vi "delete alarm comparison.vi"(8 "error in":errorcluster, 9 "compare index":i32, 10 "alarm name":string, 11 "alarms module configuration in":refnum<class "alarms module configuration.lvclass">) -> (0 "error out":errorcluster, 2 "removed channels":refnum<class "TBM channel.lvclass">[](array[class]), 3 "alarms module configuration out":refnum<class "alarms module configuration.lvclass">)   [LabVIEW 2013, in "alarms module configuration.lvclass"]
uses:
  alarms module configuration.lvclass
  <vilib>/NI/Tag Bus Module Framework/channel/TBM channel.lvclass
  alarms module configuration.lvclass/alarms module configuration.ctl
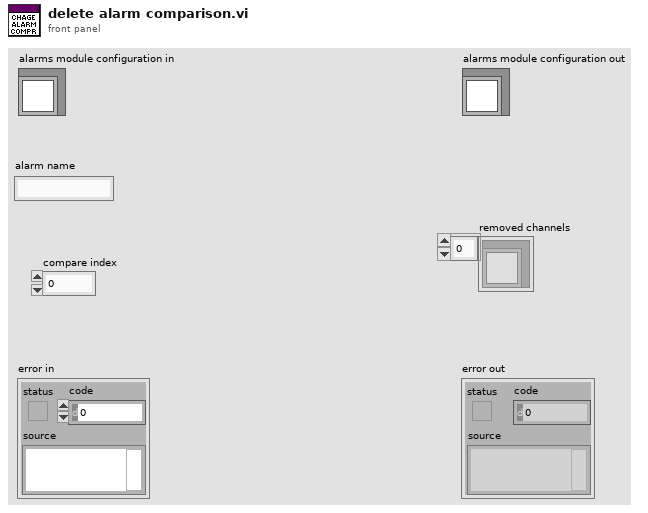
[diagram p1: front panel]
types:
  T1 = typedef "alarms module configuration.lvclass/alarm configuration.ctl" = cluster{"alarm name":string, "comparisons":T2[], "unlatch":refnum<class "TBM channel.lvclass">, "output":refnum<class "TBM channel.lvclass">, "boolean op":T4}
  T2 = typedef "alarms module configuration.lvclass/alarm comparison.ctl" = cluster{"input channel":refnum<class "TBM channel.lvclass">, "limit":dbl, "comparison":T3}
  T3 = typedef "alarms module configuration.lvclass/compare type.ctl" = enum16{">", "<", ">=", "<=", "="}
  T4 = typedef "alarms module configuration.lvclass/boolean operation.ctl" = enum16{"AND", "OR"}
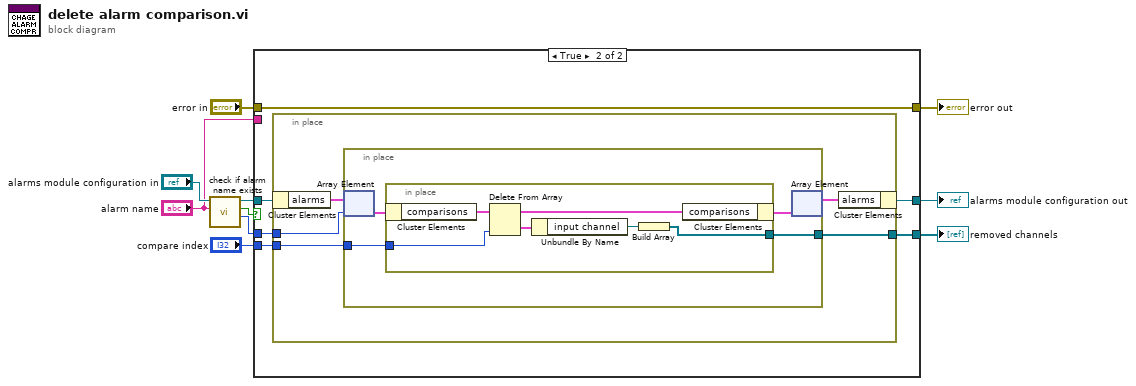
[diagram p0: block diagram]
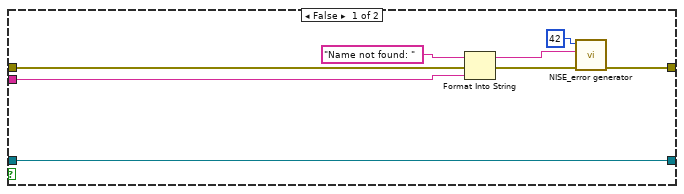
[diagram p2: hidden frame]
diagram:
  n1 = call "check if alarm name exists.vi"("name to locate"="alarm name", "alarms module configuration in"="alarms module configuration in") -> ("index"=w4:i32, "found?"=w7:bool, "alarms module configuration out"=w5:refnum<class "alarms module configuration.lvclass">)  [unwired: 6 in, 1 out]
  n2 = case shown="True" w7 {
    tunnel: [w17 w22] -> w9
    tunnel: "error in" -> [w18 w22]
    tunnel: [w12 w23] -> w6
    tunnel: w5 -> [w12 w24]
    tunnel: w4 -> [_ w21]
    tunnel: "alarm name" -> [w11 _]
    tunnel: "compare index" -> [_ w20]
    tunnel: [_ w19] -> w1
    frame False {
      n3 = Format Into String(initial string="Name not found: " ("append error message"), error in=w18, w11) -> (resulting string=w13:string, error out=w15:errorcluster)  [unwired: 1 in]
      n4 = call <vilib>:"NISE_error generator.vi"("error in"=w15, "append error message"=w13, "error code (0)"=42) -> ("error out"=w17:errorcluster)  [unwired: 6 in]
    }
    frame True {
      n5 = in-place {
        in-place-border: w21 -> [w27]
        in-place-border: w20 -> [w26]
        in-place-border: [w25] -> w19
        n6 = in-place-cluster #1(w24) -> ("alarms"=w29:T1[])
        n7 = in-place {
          in-place-border: w26 -> [w31]
          in-place-border: [w30] -> w25
          n8 = in-place-array #2(w29, w27) -> (w33:T1)
          n9 = in-place {
            in-place-border: w31 -> [w37]
            in-place-border: [w34] -> w30
            n10 = in-place-cluster #3(w33) -> ("comparisons"=w39:T2[])
            n11 = Delete From Array(array=w39, index=w37) -> (deleted portion=w36:T2, array with subset deleted=w38:T2[])  [unwired: 1 in]
            n12 = Unbundle By Name(w36) -> ("input channel"=w35:refnum<class "TBM channel.lvclass">)
            n13 = Build Array(w35) -> (w34:refnum<class "TBM channel.lvclass">[])
            n14 = in-place-cluster #3("comparisons"=w38) -> (w32:T1)
          }
          n15 = in-place-array #2(w32) -> (w28:T1[])  [unwired: 1 out]
        }
        n16 = in-place-cluster #1("alarms"=w28) -> (w23:refnum<class "alarms module configuration.lvclass">)
      }
    }
  }
  "error out" <- w9
  "alarms module configuration out" <- w6
  "removed channels" <- w1
